vi "FMA1600A Update Meter Accuracy.vi"(5 "Full Scale Index":i32, 7 "Reading Index":i32, 8 "Error In":errorcluster, 10 "Meter Accuracy Option 1":T1, 11 "Start Up File in in":string[][](array[string])) -> (0 "Error Out":errorcluster, 3 "Start Up File out":string[][](array[string]))   [LabVIEW 2023]
uses:
  Type Definitions/FMA1600A Meter Accuracy Options.ctl
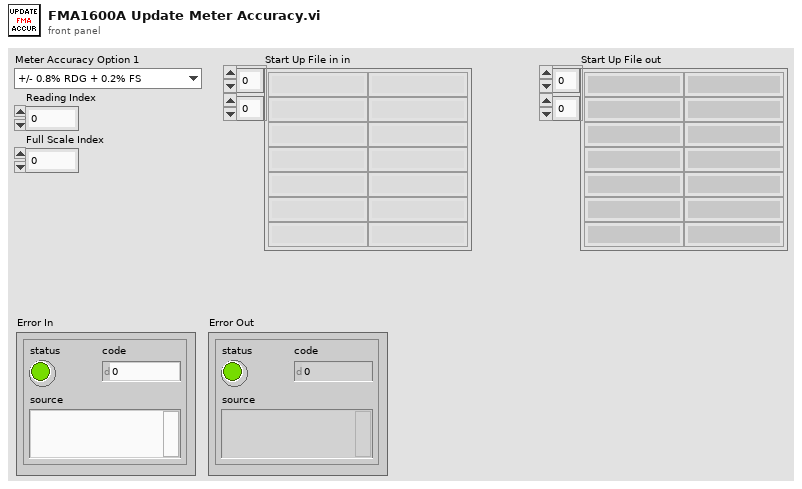
[diagram p1: front panel]
types:
  T1 = typedef "FMA1600A Meter Accuracy Options.ctl" = enum16{"+/- 0.8% RDG + 0.2% FS", "+/- 0.4% RDG + 0.2% FS"}
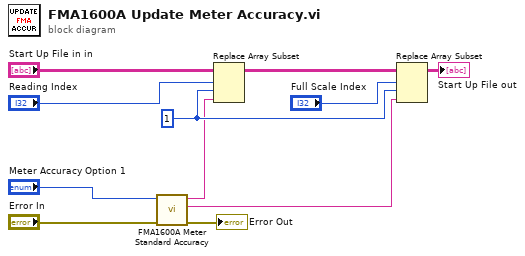
[diagram p0: block diagram]
diagram:
  w10 = 1 ("disabled index (col)")
  n1 = call "FMA1600A Meter Standard Accuracy.vi"("Error In"="Error In", "Meter Accuracy Option 1"="Meter Accuracy Option 1") -> ("Error Out"=→"Error Out":errorcluster, "Full Scale Accuracy %"=w3:string, "Reading Accuracy %"=w4:string)  [unwired: 7 in]
  n2 = Replace Array Subset(array="Start Up File in in", new element=w4, index (row)="Reading Index", index (col)=w10) -> (w8:string[][])
  n3 = Replace Array Subset(array=w8, new element=w3, index (row)="Full Scale Index", index (col)=w10) -> (→"Start Up File out":string[][])
